vi "SVT Spurious Free Dynamic Range (Frequency) (1 Ch).vi"(0 "complex spectrum":T9={"complex spectrum response"={"f0"=0.0, "df"=1.0, "complex spectrum"=[]}, "spectrum info"={"channel name"="", "description"="", "x-axis units"=0, "spectral info"={"spectrum type"=enum."Power [Magnitude^2]", "linear/dB"=enum."linear", "window"=0, "window size"=0, "FFT size"=0}, "engineering units"=0, "custom label"="", "dB reference [EU]"=0.0, "peak units"=enum."rms", "weighting filter"=0, "spectral density?"=FALSE, "unit label"="", "spectrum skewed?"=FALSE, "complimentary spectrum units"=enum."none"}} {"spectrum info"."x-axis units" items=["Time (s)"=0, "Frequency-CB (Hz)"=1, "Frequency-CPB (Hz)"=1248, "Frequency-Arbitrary (Hz)"=2357, "Quefrency (s)"=2, "Revolutions (rev)"=3, "Order"=4, "Speed (RPM)"=11, "Speed (rad/s)"=21, "Index"=65535]; "spectrum info"."weighting filter" items=["Linear", "A-weighting", "B-weighting", "C-weighting", "ITU-R 468-4", "Dolby", "CCITT", "C-message", "Wb", "Wc", "Wd", "We", "Wf", "Wh", "Wj", "Wk", "Wm", "AES17 20 kHz lowpass", "AES17 40 kHz lowpass", "AES17 20 kHz highpass", "AES17 40 kHz highpass"]; "spectrum info"."dB reference [EU]" format="%.2f"; "spectrum info"."engineering units" items=["custom..."=0, "V"=1, "A"=21, "C"=30, "pC"=31, "s"=32, "-"=29, "Pa"=2, "N"=20, "g"=3, "m/s^2"=4, "m/s"=5, "m"=6, "mm/s"=12, "mm"=13, "micron/s"=14, "micron"=15, "in/s^2"=7, "in/s"=8, "in"=9, "mil/s"=10, "mil"=11, "rad/s^2"=16, "rad/s"=17, "rad"=18, "deg/s^2"=26, "deg/s"=27, "deg"=28, "RPM"=22, "cycle/s^2"=23, "Hz"=24, "cycle"=25, "strain"=19]; "spectrum info"."spectral info"."window" items=["None "=0, "Hanning"=1, "Hamming"=2, "Blackman-Harris"=3, "Exact Blackman"=4, "Blackman"=5, "Flat Top"=6, "4 Term B-Harris "=7, "7 Term B-Harris"=8, "Low Sidelobe"=9, "Force - Exponential"=10, "Gaussian"=62]; "complex spectrum response"."complex spectrum" format="%.2f"; "complex spectrum response"."df" format="%.2f"; "complex spectrum response"."f0" format="%.2f"}, 2 "frequency range":T10={"start frequency"=-1.0, "stop frequency"=-1.0} {"stop frequency" format="%.2f"; "start frequency" format="%.2f"}, 3 "advanced span [Hz]":dbl=-1.0 format="%.2f", 4 "threshold [dBc]":dbl=inf format="%.2f", 5 "error in (no error)":errorcluster, 6 "desired units":T2={"spurious free dynamic range units"=enum."dB", "detected fundamental amplitude units"=enum."EU peak", "dB reference for detected peaks"=enum."dB ref"}, 7 "exclude harmonics":bool, 9 "expected fundamental\nfrequency [Hz]":dbl=-1.0 format="%.2f") -> (11 "detected fundamental\nfrequency [Hz]":dbl=nan format="%.2f", 12 "unit labels":T1, 13 "detected fundamental\namplitude":dbl=nan format="%.2f", 14 "complex spectrum":T9={"complex spectrum response"={"f0"=0.0, "df"=1.0, "complex spectrum"=[]}, "spectrum info"={"channel name"="", "description"="", "x-axis units"=0, "spectral info"={"spectrum type"=enum."Power [Magnitude^2]", "linear/dB"=enum."linear", "window"=0, "window size"=0, "FFT size"=0}, "engineering units"=0, "custom label"="", "dB reference [EU]"=0.0, "peak units"=enum."rms", "weighting filter"=0, "spectral density?"=FALSE, "unit label"="", "spectrum skewed?"=FALSE, "complimentary spectrum units"=enum."none"}} {"spectrum info"."x-axis units" items=["Time (s)"=0, "Frequency-CB (Hz)"=1, "Frequency-CPB (Hz)"=1248, "Frequency-Arbitrary (Hz)"=2357, "Quefrency (s)"=2, "Revolutions (rev)"=3, "Order"=4, "Speed (RPM)"=11, "Speed (rad/s)"=21, "Index"=65535]; "spectrum info"."weighting filter" items=["Linear", "A-weighting", "B-weighting", "C-weighting", "ITU-R 468-4", "Dolby", "CCITT", "C-message", "Wb", "Wc", "Wd", "We", "Wf", "Wh", "Wj", "Wk", "Wm", "AES17 20 kHz lowpass", "AES17 40 kHz lowpass", "AES17 20 kHz highpass", "AES17 40 kHz highpass"]; "spectrum info"."dB reference [EU]" format="%.2f"; "spectrum info"."engineering units" items=["custom..."=0, "V"=1, "A"=21, "C"=30, "pC"=31, "s"=32, "-"=29, "Pa"=2, "N"=20, "g"=3, "m/s^2"=4, "m/s"=5, "m"=6, "mm/s"=12, "mm"=13, "micron/s"=14, "micron"=15, "in/s^2"=7, "in/s"=8, "in"=9, "mil/s"=10, "mil"=11, "rad/s^2"=16, "rad/s"=17, "rad"=18, "deg/s^2"=26, "deg/s"=27, "deg"=28, "RPM"=22, "cycle/s^2"=23, "Hz"=24, "cycle"=25, "strain"=19]; "spectrum info"."spectral info"."window" items=["None "=0, "Hanning"=1, "Hamming"=2, "Blackman-Harris"=3, "Exact Blackman"=4, "Blackman"=5, "Flat Top"=6, "4 Term B-Harris "=7, "7 Term B-Harris"=8, "Low Sidelobe"=9, "Force - Exponential"=10, "Gaussian"=62]; "complex spectrum response"."complex spectrum" format="%.2f"; "complex spectrum response"."df" format="%.2f"; "complex spectrum response"."f0" format="%.2f"}, 16 "spurious free dynamic range":dbl=nan format="%.2f", 17 "detected peaks":cluster{"frequency [Hz]":dbl, "amplitude":dbl}[](array[cluster]) {"amplitude" format="%.2f"; "frequency [Hz]" format="%.2f"}, 18 "index of highest spur":i32, 19 "error out":errorcluster)   [LabVIEW 2017, in "SoundVib_SingleTone.lvlib"]
doc: "Computes the spurious-free dynamic range (SFDR) of <B>scaled signal</B> and returns the detected fundamental frequency, detected fundamental amplitude, spurious free dynamic range, and all detected peaks. Wire data to the <B>scaled signal [EU]</B> input to determine the polymorphic instance to use or manually select the instance."
uses:
  <vilib>/addons/Sound and Vibration/svt_Single Tone Measurements/SoundVib_SingleTone.lvlib
  <vilib>/addons/_NISVFA/_Shared subVIs/Controls/svc_Spectrum Info.ctl
  <vilib>/addons/_NISVFA/_Shared subVIs/Controls/svc_X-Axis Units.ctl
  <vilib>/addons/_NISVFA/_Shared subVIs/Controls/svc_Spectrum Type.ctl
  <vilib>/addons/_NISVFA/_Shared subVIs/Controls/svc_Engineering Units Text Ring.ctl
  <vilib>/addons/_NISVFA/_Shared subVIs/Controls/svc_Weighting Filter Text Ring.ctl
  <vilib>/addons/_NISVFA/_Shared subVIs/Controls/svc_Complimentary Spectrum Units.ctl
  <vilib>/addons/_NISVFA/_Spectrum Processing/SVFA Spectrum Peak Search (1 Ch).vi
  <vilib>/addons/_NISVFA/_Spectrum Processing/subVIs/svfa_Spectrum Peak Search.vi
  <vilib>/addons/_NISVFA/_Spectrum Processing/subVIs/svfa_Peak Rough Search Indices.vi
  <vilib>/addons/_NISVFA/_Shared subVIs/Common/svc_Get Weighting Enum and Labels.vi
  <vilib>/addons/_NISVFA/_Shared subVIs/Common/svc_Unit Label Lexical Class.vi
  <vilib>/addons/_NISVFA/_Shared subVIs/Common/svc_Engineering Units to Unit Label.vi
  <vilib>/addons/_NISVFA/_Shared subVIs/Common/svc_Format Value (DBL).vi
  <vilib>/addons/_NISVFA/_Spectrum Processing/subVIs/svfa_Three Finger Peak Search.vi
  <vilib>/addons/_NISVFA/_Spectrum Processing/SVFA Unit Conversion (Complex) (1 Ch).vi
  <vilib>/addons/_NISVFA/_Spectrum Processing/SVFA Get Spectrum Subset (Complex) (1 Ch).vi
  <vilib>/addons/Sound and Vibration/svt_Distortion/SoundVib_Distortion.lvlib
  <vilib>/Analysis/NI_AALBase.lvlib
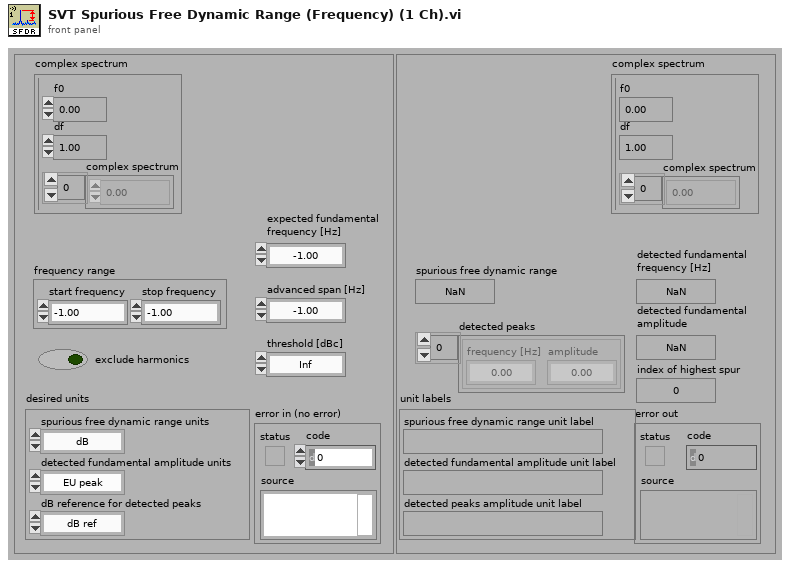
[diagram p1: front panel]
types:
  T1 = cluster{"spurious free dynamic range unit label":string, "detected fundamental amplitude unit label":string, "detected peaks amplitude unit label":string}
  T2 = cluster{"spurious free dynamic range units":enum16{"dB", "ENOB"}, "detected fundamental amplitude units":enum16{"EU rms", "EU peak", "EU peak-peak"}, "dB reference for detected peaks":enum16{"fundamental", "dB ref"}}
  T3 = typedef "svc_Spectrum Info.ctl" = cluster{"channel name":string, "description":string, "x-axis units":T4, "spectral info":cluster{"spectrum type":T5, "linear/dB":enum16{"linear", "dB"}, "window":u16, "window size":i32, "FFT size":i32}, "engineering units":T6, "custom label":string, "dB reference [EU]":dbl, "peak units":enum16{"rms", "peak", "peak-peak"}, "weighting filter":T7, "spectral density?":bool, "unit label":string, "spectrum skewed?":bool, "complimentary spectrum units":T8}
  T4 = typedef "svc_X-Axis Units.ctl" = u16
  T5 = typedef "svc_Spectrum Type.ctl" = enum16{"FFT Spectrum [complex]", "Amplitude [Magnitude]", "Power [Magnitude^2]", "Cross Spectrum [complex]", "Frequency Response [Complex]"}
  T6 = typedef "svc_Engineering Units Text Ring.ctl" = u16
  T7 = typedef "svc_Weighting Filter Text Ring.ctl" = u16
  T8 = typedef "svc_Complimentary Spectrum Units.ctl" = enum16{"none", "radians", "degrees", "cycles", "imaginary"}
  T9 = cluster{"complex spectrum response":cluster{"f0":dbl, "df":dbl, "complex spectrum":cdb[]}, "spectrum info":T3}
  T10 = cluster{"start frequency":dbl, "stop frequency":dbl}
  T11 = cluster{"single/multiple":enum16{"Multiple Peaks", "Single Max Peak"}, "threshold":dbl}
  T12 = cluster{"linear/dB":enum16{"no change", "linear", "dB"}, "dB reference (0: no change)":dbl, "power/magnitude":enum16{"no change", "power", "magnitude"}, "view":enum16{"no change", "rms", "peak", "peak-peak"}}
  T13 = enum16{"none", "input signal", "detected signal", "residual signal"}
  T14 = cluster{"complex spectrum subset":cluster{"x0":dbl, "dx":dbl, "complex array":cdb[]}, "spectrum info":T3}
  T15 = cluster{string, "unit label":string, "unit label":string}
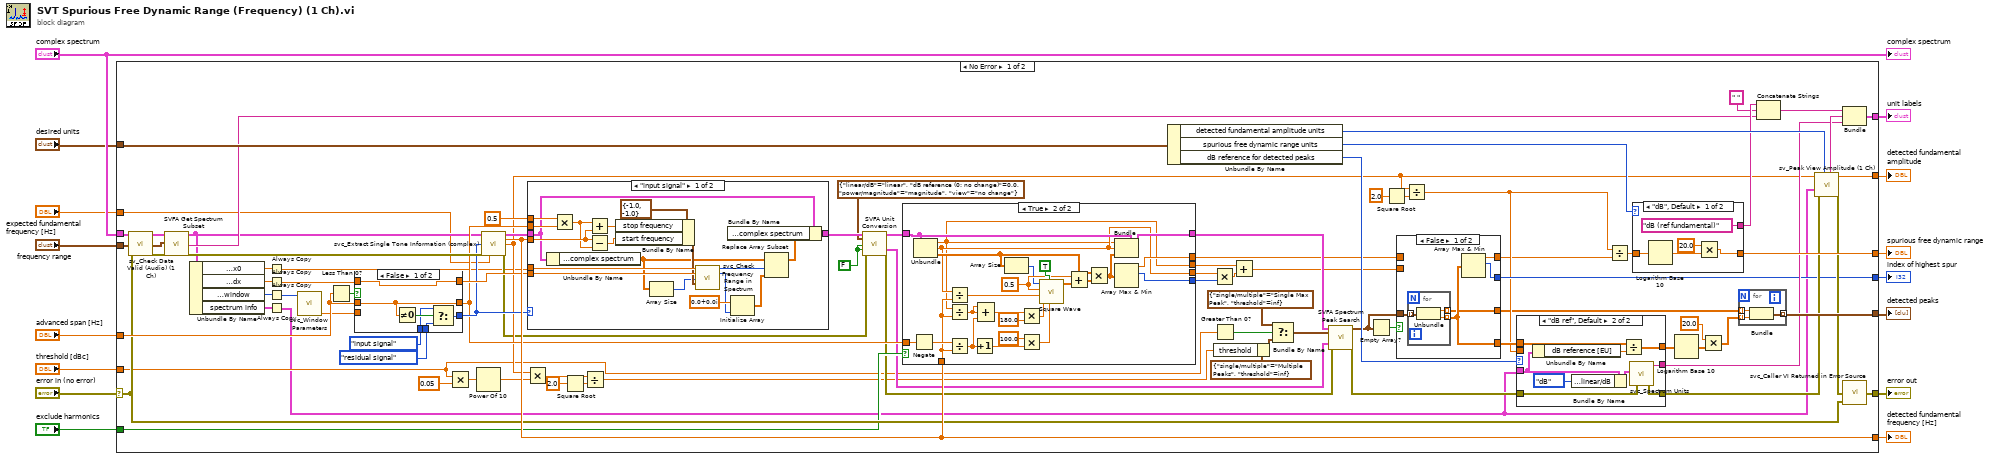
[diagram p0: block diagram]
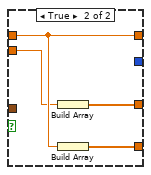
[diagram p2: hidden frame]
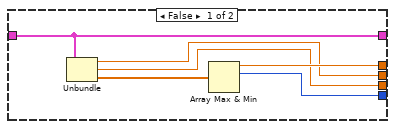
[diagram p3: hidden frame]
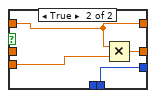
[diagram p5: hidden frame]
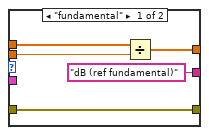
[diagram p6: hidden frame]
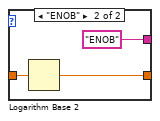
[diagram p7: hidden frame]
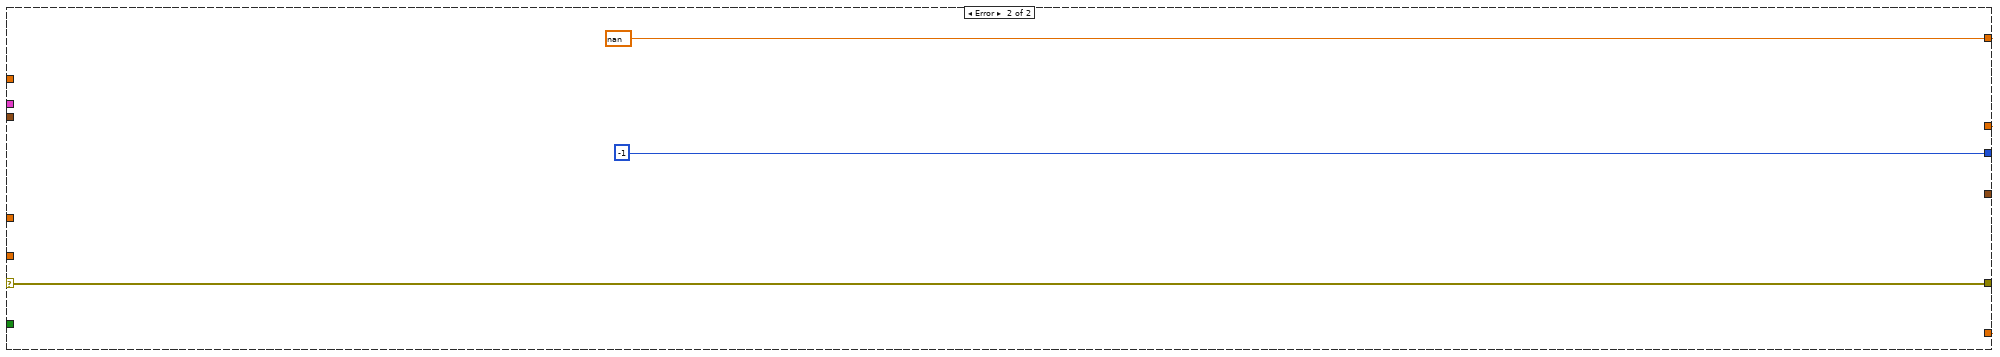
[diagram p8: hidden frame]
diagram:
  n1 = case shown="No Error" "error in (no error)" {
    selector: "error in (no error)" -> [w83 w205]
    tunnel: "complex spectrum" -> [w64 _]
    tunnel: "frequency range" -> [w92 _]
    tunnel: [w96 w205] -> w14
    tunnel: [w100 w204] -> w13
    tunnel: [w97 _] -> w10
    tunnel: [w104 w204] -> w8
    tunnel: [w85 w204] -> w9
    tunnel: "desired units" -> [w103 _]
    tunnel: [w98 _] -> w6
    tunnel: [w47 -1] -> w5
    tunnel: "advanced span [Hz]" -> [w84 _]
    tunnel: "exclude harmonics" -> [w65 _]
    tunnel: "threshold [dBc]" -> [w32 _]
    tunnel: "expected fundamental\nfrequency [Hz]" -> [w31 _]
    frame No Error {
      w67 = FALSE ("convert to degree (T)")
      n2 = call <vilib>:"sv_Check Data Valid (Audio) (1 Ch).vi"("complex spectrum"=w64, "frequency range in"=w92, "error in (no error)"=w83) -> ("complex spectrum"=w82:T9, "frequency range out"=w87:T10, "error out"=w81:errorcluster)  [unwired: 9 in, 5 out]
      n3 = call-poly <vilib>:"SVFA Get Spectrum Subset.vi"("complex spectrum"=w82, "range"=w87, "error in (no error)"=w81) -> ("complex spectrum subset"=w57:T14, "range label"=w86:string, "error out"=w80:errorcluster)  [unwired: 13 in, 1 out]
      n4 = Unbundle By Name(w57) -> ("complex spectrum subset.x0"=w76:dbl, "complex spectrum subset.dx"=w70:dbl, "spectrum info.spectral info.window"=w78:u16, "spectrum info"=w63:T3)
      n5 = Always Copy(1:w76) -> (0:w30:dbl)
      n6 = Always Copy(1:w70) -> (0:w29:dbl)
      n7 = Always Copy(1:w78) -> (0:w28:u16)
      n8 = Always Copy(1:w63) -> (0:w26:T3)
      n9 = call <vilib>:"svc_Window Parameters.vi"("window"=w28) -> ("maximum BW"=w27:dbl)  [unwired: 7 in, 3 out]
      n10 = Less Than 0?(x=w84) -> (x < 0?=w79:bool)
      n11 = case shown="False" w79 {
        tunnel: [w173 w177] -> w58
        tunnel: w84 -> [w173 _]
        tunnel: w29 -> [w168 w175]
        tunnel: T13."input signal" ("export signals") -> [w171 _]
        tunnel: T13."residual signal" ("export signals") -> [w170 w176]
        tunnel: [w169 w176] -> w74
        tunnel: [w168 w175] -> w75
        tunnel: w27 -> [_ w174]
        frame False {
          n12 = Not Equal To 0?(x=w173) -> (x != 0?=w172:bool)
          n13 = Select(t=w171, s=w172, f=w170) -> (s? t:f=w169:T13)
        }
        frame True {
          n14 = Multiply(x=w175, y=w174) -> (x*y=w177:dbl)
        }
      }
      n15 = Multiply(x=w32, y=0.05) -> (x*y=w45:dbl)
      n16 = Power Of 10(x=w45) -> (10^x=w44:dbl)
      n17 = call <vilib>:"svc_Extract Single Tone Information (complex).vi"("complex spectrum"=w57, "export signals"=w74, "error in"=w80, "approximate frequency [Hz]"=w31) -> ("complex spectrum"=w73:T9, "frequency [Hz]"=w104:dbl, "amplitude [EU pk]"=w41:dbl, "error out"=w40:errorcluster)  [unwired: 6 in, 2 out]
      n18 = Multiply(x=w41, y=w44) -> (x*y=w33:dbl)
      n19 = case shown="\"input signal\"" w74 {
        tunnel: w30 -> [w159 _]
        tunnel: w104 -> [w164 _]
        tunnel: w75 -> [w158 _]
        tunnel: w58 -> [w154 _]
        tunnel: w73 -> [w149 w167]
        tunnel: 0.5 ("value") -> [w151 _]
        tunnel: [w150 w167] -> w69
        frame "input signal" {
          n20 = Unbundle By Name(w149) -> ("complex spectrum response.complex spectrum"=w153:cdb[])
          n21 = Multiply(x=w151, y=w154) -> (x*y=w163:dbl)
          n22 = Add(x=w163, y=w164) -> (x+y=w161:dbl)
          n23 = Subtract(x=w164, y=w163) -> (x-y=w160:dbl)
          n24 = Bundle By Name(cluster=T10 {"start frequency"=-1.0, "stop frequency"=-1.0} ("frequency range"), "stop frequency"=w161, "start frequency"=w160) -> (w155:T10)
          n25 = Array Size(array=w153) -> (size(s)=w152:i32)
          n26 = call <vilib>:"svc_Check Frequency Range in Spectrum.vi"("f0"=w159, "df"=w158, "spectrum length"=w152, "frequency range"=w155) -> ("start index"=w157:i32, "band length"=w156:i32)  [unwired: 7 in, 3 out]
          n27 = Initialize Array(cdb 0.0+0.0i ("element"), w156) -> (w165:cdb[])
          n28 = Replace Array Subset(array=w153, new element=w165, index=w157) -> (w148:cdb[])
          n29 = Bundle By Name(cluster=w149, "complex spectrum response.complex spectrum"=w148) -> (w150:T9)
        }
        frame "residual signal", Default {
        }
      }
      n30 = Square Root(x=2.0 ("y")) -> (sqrt(x)=w34:dbl)
      n31 = Divide(x=w33, y=w34) -> (x/y=w24:dbl)
      n32 = call-poly <vilib>:"SVFA Unit Conversion.vi"("complex spectrum"=w69, "desired scaling"=T12 {"linear/dB"=enum."linear", "dB reference (0: no change)"=0.0, "power/magnitude"=enum."magnitude", "view"=enum."no change"}, "unwrap phase (F)"=w67, "convert to degree (T)"=w67, "error in (no error)"=w40) -> ("converted spectrum"=w66:cluster{"x0":dbl, "dx":dbl, "magnitude":dbl[]}, "spectrum info out"=w54:T3, "error out"=w56:errorcluster)  [unwired: 9 in, 3 out]
      n33 = case shown="True" w65 {
        tunnel: w66 -> [w122 w136]
        tunnel: [w122 w138] -> w48
        tunnel: w104 -> [_ w132]
        tunnel: w58 -> [_ w135]
        tunnel: [w120 w126] -> w21
        tunnel: [w119 w125] -> w19
        tunnel: [w118 w124] -> w18
        tunnel: [w117 w123] -> w17
        frame False {
          n34 = Unbundle(w122) -> ("x0"=w117:dbl, "dx"=w118:dbl, "magnitude"=w121:dbl[])
          n35 = Array Max & Min(array=w121) -> (max value=w120:dbl, max index (indices)=w119:i32)  [unwired: 2 out]
        }
        frame True {
          w141 = 0.5 ("amplitude")
          n36 = Negate(x=w135) -> (-x=w134:dbl)
          n37 = Unbundle(w136) -> ("x0"=w123:dbl, "dx"=w124:dbl, "magnitude"=w137:dbl[])
          n38 = Divide(x=w124, y=w132) -> (x/y=w133:dbl)
          n39 = Divide(x=w123, y=w132) -> (x/y=w131:dbl)
          n40 = Divide(x=w134, y=w132) -> (x/y=w130:dbl)
          n41 = Increment(x=w130) -> (x+1=w143:dbl)
          n42 = Compound Arithmetic op=ADD(w131, w131, w130) -> (w129:dbl)
          n43 = Array Size(array=w137) -> (size(s)=w140:i32)
          n44 = Multiply(x=w129, y=180.0) -> (x*y=w128:dbl)
          n45 = Multiply(x=100.0, y=w143) -> (x*y=w145:dbl)
          n46 = call <vilib>:"Square Wave.vi"("samples"=w140, "reset phase"=TRUE, "amplitude"=w141, "frequency"=w133, "duty cycle (%)"=w145, "phase in"=w128) -> ("square wave"=w146:dbl[])  [unwired: 2 out]
          n47 = Add(x=w141, y=w146) -> (x+y=w139:dbl[])
          n48 = Multiply(x=w137, y=w139) -> (x*y=w127:dbl[])
          n49 = Bundle(cluster=w136, "x0"=w123, "dx"=w124, "magnitude"=w127) -> (w138:cluster{"x0":dbl, "dx":dbl, "magnitude":dbl[]})
          n50 = Array Max & Min(array=w127) -> (max value=w126:dbl, max index (indices)=w125:i32)  [unwired: 2 out]
        }
      }
      n51 = Unbundle By Name(w103) -> ("detected fundamental amplitude units"=w102:enum16{"EU rms", "EU peak", "EU peak-peak"}, "spurious free dynamic range units"=w99:enum16{"dB", "ENOB"}, "dB reference for detected peaks"=w90:enum16{"fundamental", "dB ref"})
      n52 = Multiply(x=w18, y=w19) -> (x*y=w20:dbl)
      n53 = Greater Than 0?(x=w32) -> (x > 0?=w52:bool)
      n54 = Bundle By Name(cluster=T11 {"single/multiple"=enum."Multiple Peaks", "threshold"=inf} ("peak search settings"), "threshold"=w24) -> (w50:T11)
      n55 = Add(x=w17, y=w20) -> (x+y=w16:dbl)
      n56 = Select(t=T11 {"single/multiple"=enum."Single Max Peak", "threshold"=inf} ("peak search settings"), s=w52, f=w50) -> (s? t:f=w49:T11)
      n57 = call-poly <vilib>:"SVFA Spectrum Peak Search.vi"("spectrum"=w48, "peak search settings"=w49, "spectrum info in"=w54, "error in (no error)"=w56) -> ("peaks"=w23:cluster{"freq. or order":dbl, "value":dbl}[], "error out"=w55:errorcluster)  [unwired: 11 in, 3 out]
      n58 = Empty Array?(array=w23) -> (empty?=w22:bool)
      n59 = Square Root(x=2.0 ("y")) -> (sqrt(x)=w42:dbl)
      n60 = case shown="False" w22 {
        tunnel: [w109 _] -> w47
        tunnel: [w108 w115] -> w39
        tunnel: [w107 w116] -> w36
        tunnel: [w106 w113] -> w25
        tunnel: w23 -> [w105 _]
        tunnel: w21 -> [_ w116]
        tunnel: w16 -> [_ w114]
        frame False {
          n61 = for {
            tunnel: w105 -> [w112] mode=indexing
            tunnel: [w111] -> w106 mode=indexing
            tunnel: [w110] -> w108 mode=indexing
            n62 = Unbundle(w112) -> ("freq. or order"=w111:dbl, "value"=w110:dbl)
          }
          n63 = Array Max & Min(array=w108) -> (max value=w107:dbl, max index (indices)=w109:i32)  [unwired: 2 out]
        }
        frame True {
          n64 = Build Array(w114) -> (w113:dbl[])
          n65 = Build Array(w116) -> (w115:dbl[])
        }
      }
      n66 = Divide(x=w41, y=w42) -> (x/y=w37:dbl)
      n67 = case shown="\"dB ref\", Default" w90 {
        tunnel: w39 -> [w180 w188]
        tunnel: [w179 w183] -> w59
        tunnel: w26 -> [_ w185]
        tunnel: w55 -> [w182 w191]
        tunnel: [w182 w190] -> w89
        tunnel: ["dB (ref fundamental)" ("unit label") w189] -> w88
        tunnel: w37 -> [w178 _]
        frame "fundamental" {
          n68 = Divide(x=w180, y=w178) -> (x/y=w179:dbl[])
        }
        frame "dB ref", Default {
          n69 = Unbundle By Name(w185) -> ("dB reference [EU]"=w187:dbl)
          n70 = Bundle By Name(cluster=w185, "spectral info.linear/dB"=enum16{"linear", "dB"}."dB") -> (w184:T3)
          n71 = Divide(x=w188, y=w187) -> (x/y=w183:dbl[])
          n72 = call <vilib>:"svc_Spectrum Units.vi"("error in (no error)"=w191, "spectrum info in"=w184) -> ("error out"=w190:errorcluster, "unit label"=w189:string)  [unwired: 2 in, 2 out]
        }
      }
      n73 = Divide(x=w37, y=w36) -> (x/y=w38:dbl)
      n74 = case shown="\"dB\", Default" w99 {
        tunnel: w38 -> [w199 w202]
        tunnel: [w195 w201] -> w100
        tunnel: ["dB (ref fundamental)" ("unit label") "ENOB" ("unit label")] -> w95
        frame "dB", Default {
          n75 = Logarithm Base 10(1:w199) -> (0:w196:dbl)
          n76 = Multiply(x=20.0 ("y"), y=w196) -> (x*y=w195:dbl)
        }
        frame "ENOB" {
          n77 = Logarithm Base 2(1:w202) -> (0:w201:dbl)
        }
      }
      n78 = Logarithm Base 10(1:w59) -> (0:w61:dbl[])
      n79 = Multiply(x=20.0 ("y"), y=w61) -> (x*y=w60:dbl[])
      n80 = for {
        tunnel: w25 -> [w193] mode=indexing
        tunnel: w60 -> [w194] mode=indexing
        tunnel: [w192] -> w97 mode=indexing
        n81 = Bundle("freq. or order"=w193, w194) -> (w192:cluster{"freq. or order":dbl, dbl})  [unwired: 1 in]
      }
      n82 = Concatenate Strings(w95, " " ("string"), w86) -> (w94:string)
      n83 = call <vilib>:"sv_Peak View Amplitude (1 Ch).vi"("peak units"=w102, "error in (no error)"=w89, "spectrum info"=w26, "peak amplitude [EU pk]"=w41) -> ("error out"=w91:errorcluster, "converted peak amplitude"=w85:dbl, "unit label"=w101:string)  [unwired: 5 in]
      n84 = Bundle(w94, "unit label"=w101, "unit label"=w88) -> (w98:T15)  [unwired: 1 in]
      n85 = call <vilib>:"svc_Caller VI Returned in Error Source.vi"("warning input to caller"=w83, "error in (no error)"=w91) -> ("error out"=w96:errorcluster)  [unwired: 3 in]
    }
    frame Error {
      w204 = nan
    }
  }
  "error out" <- w14
  "spurious free dynamic range" <- w13
  "unit labels" <- w6
  "detected peaks" <- w10
  "detected fundamental\nfrequency [Hz]" <- w8
  "detected fundamental\namplitude" <- w9
  "index of highest spur" <- w5
  "complex spectrum" <- "complex spectrum"
